vi "Pre Launch Init.vi"(11 "Server in":refnum<class "Server.lvclass">) -> (0 "error out":errorcluster, 3 "Server out":refnum<class "Server.lvclass">)   [LabVIEW 2021, in "Server.lvlib" / "Server.lvclass"]
doc: "(<B>Filename</B>: Actor Framework.lvlib:Actor.lvclass:Pre Launch Init.vi)\n\nDefines behavior that occurs after the Launch Nested Actor method is invoked but before the actor's Actor Core method begins running.\n\nBy default, this method does nothing. A descendant class may override it to define behavior."
uses:
  Server.lvclass
  Server.lvclass/Server.ctl
  <vilib>/ActorFramework/Actor/Actor.lvclass
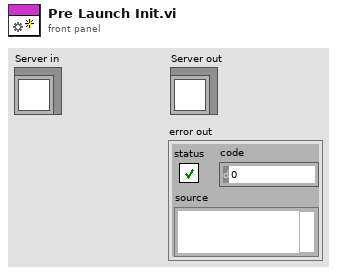
[diagram p1: front panel]
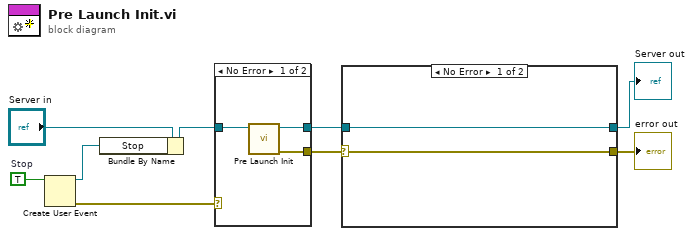
[diagram p0: block diagram]
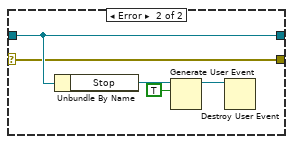
[diagram p2: hidden frame]
diagram:
  w9 = TRUE  # Stop
  n1 = Create User Event(user event datatype=w9) -> (user event=w7:refnum<user-event>, error out=w6:errorcluster)  [unwired: 1 in]
  n2 = Bundle By Name(cluster="Server in", "Stop"=w7) -> (w5:refnum<class "Server.lvclass">)
  n3 = case shown="No Error" w6 {
    selector: w6 -> [_ w13]
    tunnel: [w12 w13] -> w4
    tunnel: [w11 w14] -> w3
    tunnel: w5 -> [w10 w14]
    frame No Error {
      n4 = call-parent "Pre Launch Init.vi"("Actor in"=w10) -> ("error out"=w12:errorcluster, "Actor out"=w11:refnum<class "Server.lvclass">)  [unwired: 9 in]
    }
    frame Error {
    }
  }
  n5 = case shown="No Error" w4 {
    selector: w4 -> [w15 w17]
    tunnel: w3 -> [w16 w18]
    tunnel: [w16 w18] -> w2
    tunnel: [w15 w17] -> w1
    frame No Error {
    }
    frame Error {
      n6 = Unbundle By Name(w18) -> ("Stop"=w21:refnum<user-event>)
      n7 = Generate User Event(user event=w21, event data cluster=TRUE ("event data")) -> (user event out=w19:refnum<user-event>)  [unwired: 2 in, 1 out]
      n8 = Destroy User Event(user event=w19) -> ()  [unwired: 1 in, 1 out]
    }
  }
  "error out" <- w1
  "Server out" <- w2
